vi "fpga_LP2ControlUnit (M Class_60Hz).vi"(0 "#Ch":fxp<+,5,5>=16.0, 1 "reset":bool, 2 "input valid":bool) -> (5 "ready for input":bool, 7 "output valid":bool, 8 "opState":T1, 9 "coefRDAddr":fxp<+,11,11>)   [LabVIEW 2013, in "NI_EP_PMU_FPGA.lvlib"]
uses:
  <vilib>/addons/Electrical Power/PMU/NI_EP_PMU_FPGA.lvlib
  <vilib>/rvi/FXPMathLib/basic elements/FxpAddSub/XNode/nifxpmath_AddSub.xnode
  <vilib>/rvi/FXPMathLib/sim/FxpSim.dll
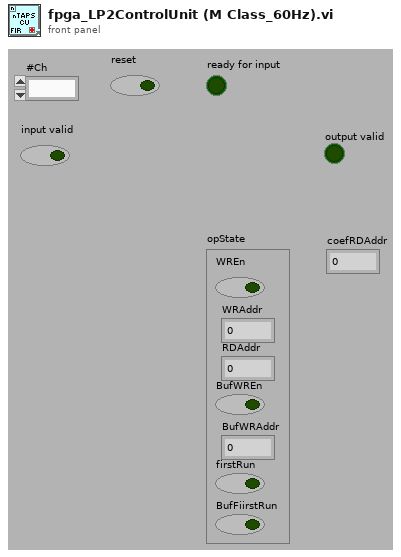
[diagram p1: front panel]
types:
  T1 = cluster{"WREn":bool, "WRAddr":fxp<+,15,15>, "RDAddr":fxp<+,15,15>, "BufWREn":bool, "BufWRAddr":fxp<+,15,15>, "firstRun":bool, "BufFiirstRun":bool}
  T2 = cluster{"idle":bool, "ready for input":bool, "macWrap":bool, "inputBufWRAddr":fxp<+,15,15>, "coefRDAddr":fxp<+,11,11>, "stateMemRDAddr":fxp<+,15,15>, "stateMemPageRDAddr":fxp<+,15,15>, "chCnt":fxp<+,5,5>, "first run?":bool, "firstRunCnt":fxp<+,15,15>, "buf first run?":bool, "bufFirstRunCnt":fxp<+,15,15>}
  T3 = cluster{"inputBufWRAddr":fxp<+,15,15>, "coefRDAddr":fxp<+,11,11>, "stateMemPageRDAddr":fxp<+,15,15>, "#Ch*(#TPPM-1)-1":fxp<+,15,15>, "#Ch*(#TPPM-2)-1":fxp<+,15,15>, "#Ch*#BufSize":fxp<+,15,15>, "2*#Ch-1":fxp<+,5,5>, "-#Ch":fxp<+,15,15>}
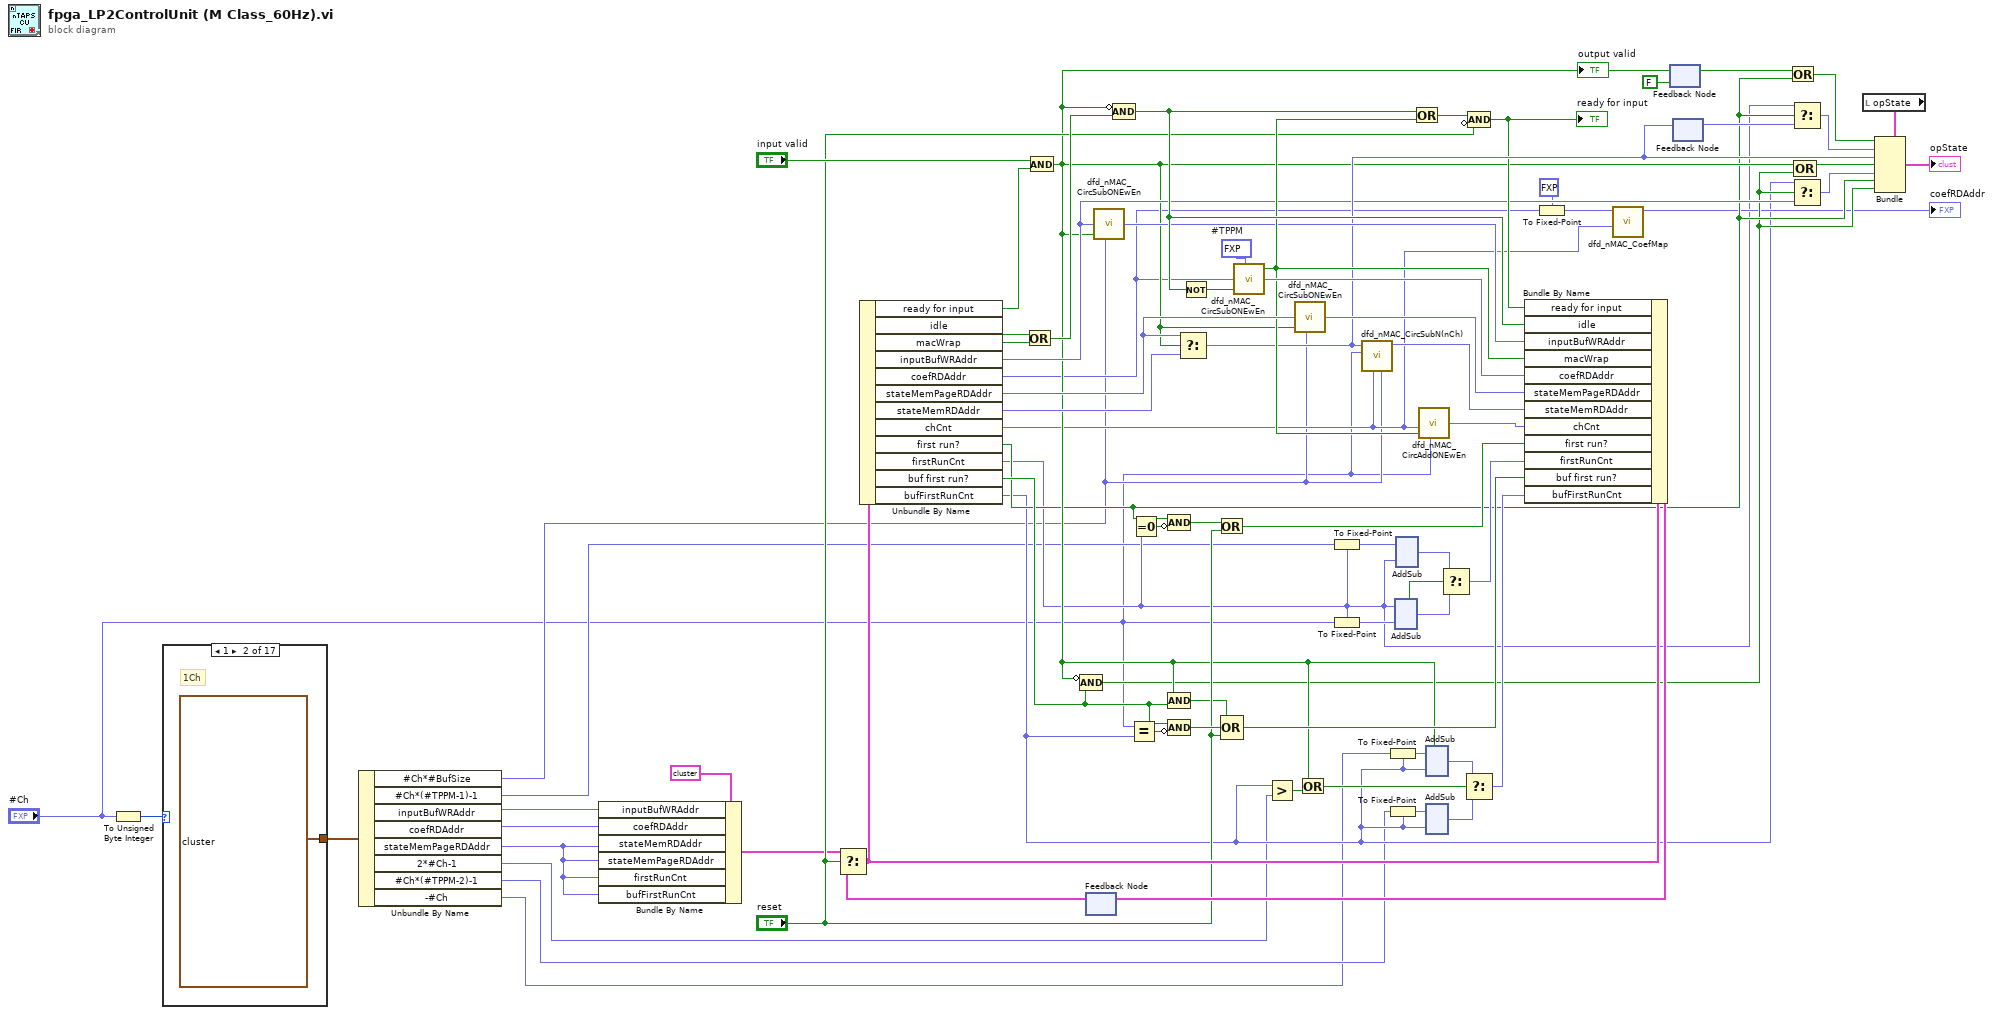
[diagram p0: block diagram]
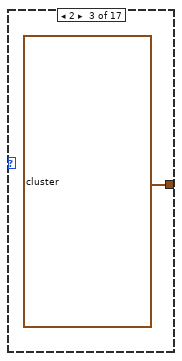
[diagram p3: hidden frame]
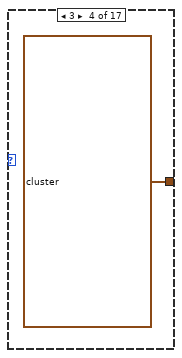
[diagram p4: hidden frame]
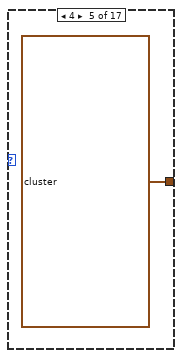
[diagram p5: hidden frame]
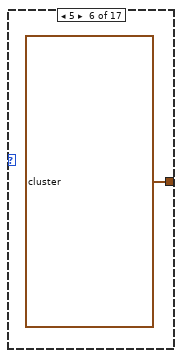
[diagram p6: hidden frame]
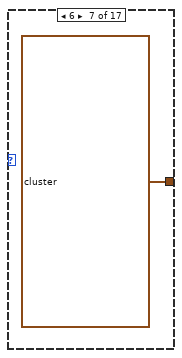
[diagram p7: hidden frame]
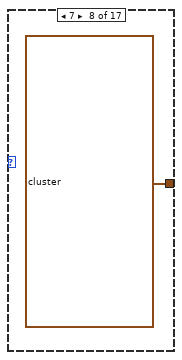
[diagram p8: hidden frame]
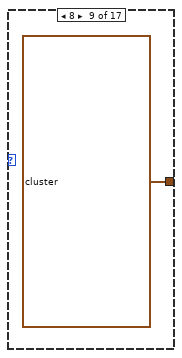
[diagram p9: hidden frame]
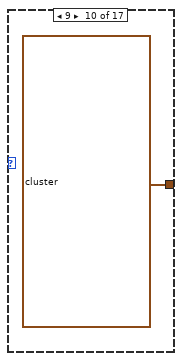
[diagram p10: hidden frame]
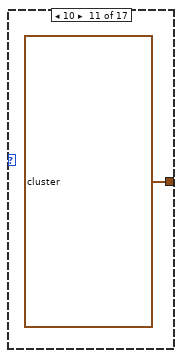
[diagram p11: hidden frame]
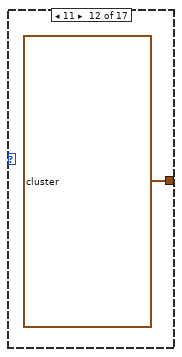
[diagram p12: hidden frame]
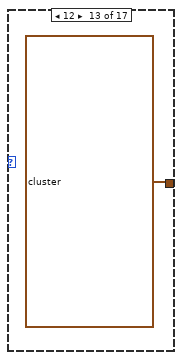
[diagram p13: hidden frame]
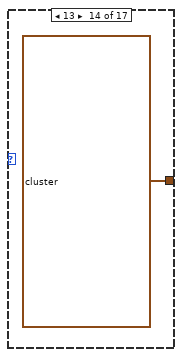
[diagram p14: hidden frame]
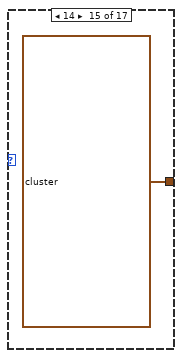
[diagram p15: hidden frame]
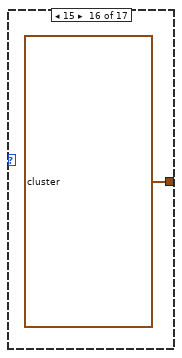
[diagram p16: hidden frame]
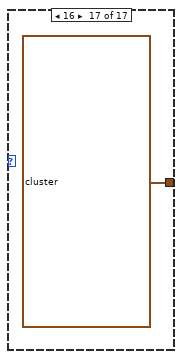
[diagram p17: hidden frame]
diagram:
  w68 = fxp<+,11,11> 1188.0  # #TPPM
  n1 = To Unsigned Byte Integer(number="#Ch") -> (unsigned 8bit integer=w13:u8)
  n2 = case shown="1" w13 {
    tunnel: [_ T3 {"inputBufWRAddr"=0.0, "coefRDAddr"=1187.0, "stateMemPageRDAddr"=1187.0, "#Ch*(#TPPM-1)-1"=1186.0, "#Ch*(#TPPM-2)-1"=1185.0, "#Ch*#BufSize"=1188.0, "2*#Ch-1"=1.0, "-#Ch"=32767.0} ("Cluster") T3 {"inputBufWRAddr"=1.0, "coefRDAddr"=1187.0, "stateMemPageRDAddr"=2375.0, "#Ch*(#TPPM-1)-1"=2373.0, "#Ch*(#TPPM-2)-1"=2371.0, "#Ch*#BufSize"=2376.0, "2*#Ch-1"=3.0, "-#Ch"=32766.0} ("Cluster") T3 {"inputBufWRAddr"=2.0, "coefRDAddr"=1187.0, "stateMemPageRDAddr"=3563.0, "#Ch*(#TPPM-1)-1"=3560.0, "#Ch*(#TPPM-2)-1"=3557.0, "#Ch*#BufSize"=3564.0, "2*#Ch-1"=5.0, "-#Ch"=32765.0} ("Cluster") T3 {"inputBufWRAddr"=3.0, "coefRDAddr"=1187.0, "stateMemPageRDAddr"=4751.0, "#Ch*(#TPPM-1)-1"=4747.0, "#Ch*(#TPPM-2)-1"=4743.0, "#Ch*#BufSize"=4752.0, "2*#Ch-1"=7.0, "-#Ch"=32764.0} ("Cluster") T3 {"inputBufWRAddr"=4.0, "coefRDAddr"=1187.0, "stateMemPageRDAddr"=5939.0, "#Ch*(#TPPM-1)-1"=5934.0, "#Ch*(#TPPM-2)-1"=5929.0, "#Ch*#BufSize"=5940.0, "2*#Ch-1"=9.0, "-#Ch"=32763.0} ("Cluster") T3 {"inputBufWRAddr"=5.0, "coefRDAddr"=1187.0, "stateMemPageRDAddr"=7127.0, "#Ch*(#TPPM-1)-1"=7121.0, "#Ch*(#TPPM-2)-1"=7115.0, "#Ch*#BufSize"=7128.0, "2*#Ch-1"=11.0, "-#Ch"=32762.0} ("Cluster") T3 {"inputBufWRAddr"=6.0, "coefRDAddr"=1187.0, "stateMemPageRDAddr"=8315.0, "#Ch*(#TPPM-1)-1"=8308.0, "#Ch*(#TPPM-2)-1"=8301.0, "#Ch*#BufSize"=8316.0, "2*#Ch-1"=13.0, "-#Ch"=32761.0} ("Cluster") T3 {"inputBufWRAddr"=7.0, "coefRDAddr"=1187.0, "stateMemPageRDAddr"=9503.0, "#Ch*(#TPPM-1)-1"=9495.0, "#Ch*(#TPPM-2)-1"=9487.0, "#Ch*#BufSize"=9504.0, "2*#Ch-1"=15.0, "-#Ch"=32760.0} ("Cluster") T3 {"inputBufWRAddr"=8.0, "coefRDAddr"=1187.0, "stateMemPageRDAddr"=10691.0, "#Ch*(#TPPM-1)-1"=10682.0, "#Ch*(#TPPM-2)-1"=10673.0, "#Ch*#BufSize"=10692.0, "2*#Ch-1"=17.0, "-#Ch"=32759.0} ("Cluster") T3 {"inputBufWRAddr"=9.0, "coefRDAddr"=1187.0, "stateMemPageRDAddr"=11879.0, "#Ch*(#TPPM-1)-1"=11869.0, "#Ch*(#TPPM-2)-1"=11859.0, "#Ch*#BufSize"=11880.0, "2*#Ch-1"=19.0, "-#Ch"=32758.0} ("Cluster") T3 {"inputBufWRAddr"=10.0, "coefRDAddr"=1187.0, "stateMemPageRDAddr"=13067.0, "#Ch*(#TPPM-1)-1"=13056.0, "#Ch*(#TPPM-2)-1"=13045.0, "#Ch*#BufSize"=13068.0, "2*#Ch-1"=21.0, "-#Ch"=32757.0} ("Cluster") T3 {"inputBufWRAddr"=11.0, "coefRDAddr"=1187.0, "stateMemPageRDAddr"=14255.0, "#Ch*(#TPPM-1)-1"=14243.0, "#Ch*(#TPPM-2)-1"=14231.0, "#Ch*#BufSize"=14256.0, "2*#Ch-1"=23.0, "-#Ch"=32756.0} ("Cluster") T3 {"inputBufWRAddr"=12.0, "coefRDAddr"=1187.0, "stateMemPageRDAddr"=15443.0, "#Ch*(#TPPM-1)-1"=15430.0, "#Ch*(#TPPM-2)-1"=15417.0, "#Ch*#BufSize"=15444.0, "2*#Ch-1"=25.0, "-#Ch"=32755.0} ("Cluster") T3 {"inputBufWRAddr"=13.0, "coefRDAddr"=1187.0, "stateMemPageRDAddr"=16631.0, "#Ch*(#TPPM-1)-1"=16617.0, "#Ch*(#TPPM-2)-1"=16603.0, "#Ch*#BufSize"=16632.0, "2*#Ch-1"=27.0, "-#Ch"=32754.0} ("Cluster") T3 {"inputBufWRAddr"=14.0, "coefRDAddr"=1187.0, "stateMemPageRDAddr"=17819.0, "#Ch*(#TPPM-1)-1"=17804.0, "#Ch*(#TPPM-2)-1"=17789.0, "#Ch*#BufSize"=17820.0, "2*#Ch-1"=29.0, "-#Ch"=32753.0} ("Cluster") T3 {"inputBufWRAddr"=15.0, "coefRDAddr"=1187.0, "stateMemPageRDAddr"=19007.0, "#Ch*(#TPPM-1)-1"=18991.0, "#Ch*(#TPPM-2)-1"=18975.0, "#Ch*#BufSize"=19008.0, "2*#Ch-1"=31.0, "-#Ch"=32752.0} ("Cluster")] -> w12
    frame 0, Default {
    }
    frame 1 {
      # "1Ch"
    }
    frame 2 {
    }
    frame 3 {
    }
    frame 4 {
    }
    frame 5 {
    }
    frame 6 {
    }
    frame 7 {
    }
    frame 8 {
    }
    frame 9 {
    }
    frame 10 {
    }
    frame 11 {
    }
    frame 12 {
    }
    frame 13 {
    }
    frame 14 {
    }
    frame 15 {
    }
    frame 16 {
    }
  }
  n3 = Unbundle By Name(w12) -> ("#Ch*#BufSize"=w6:fxp<+,15,15>, "#Ch*(#TPPM-1)-1"=w5:fxp<+,15,15>, "inputBufWRAddr"=w11:fxp<+,15,15>, "coefRDAddr"=w10:fxp<+,11,11>, "stateMemPageRDAddr"=w9:fxp<+,15,15>, "2*#Ch-1"=w4:fxp<+,5,5>, "#Ch*(#TPPM-2)-1"=w3:fxp<+,15,15>, "-#Ch"=w2:fxp<+,15,15>)
  n4 = Bundle By Name(cluster=T2 {"idle"=TRUE, "ready for input"=FALSE, "macWrap"=FALSE, "inputBufWRAddr"=15.0, "coefRDAddr"=1187.0, "stateMemRDAddr"=19007.0, "stateMemPageRDAddr"=19007.0, "chCnt"=0.0, "first run?"=TRUE, "firstRunCnt"=19007.0, "buf first run?"=TRUE, "bufFirstRunCnt"=19007.0} ("CUInitialState"), "inputBufWRAddr"=w11, "coefRDAddr"=w10, "stateMemRDAddr"=w9, "stateMemPageRDAddr"=w9, "firstRunCnt"=w9, "bufFirstRunCnt"=w9) -> (w7:T2)
  n5 = feedback #1() -> (w69:T2)  [unwired: 1 out]
  n6 = Select(t=w7, s="reset", f=w69) -> (s? t:f=w66:T2)
  n7 = Unbundle By Name(w66) -> ("ready for input"=w64:bool, "idle"=w56:bool, "macWrap"=w57:bool, "inputBufWRAddr"=w43:fxp<+,15,15>, "coefRDAddr"=w21:fxp<+,11,11>, "stateMemPageRDAddr"=w72:fxp<+,15,15>, "stateMemRDAddr"=w73:fxp<+,15,15>, "chCnt"=w23:fxp<+,5,5>, "first run?"=w26:bool, "firstRunCnt"=w17:fxp<+,15,15>, "buf first run?"=w29:bool, "bufFirstRunCnt"=w14:fxp<+,15,15>)
  n8 = Or(x=w56, y=w57) -> (x .or. y?=w63:bool)
  n9 = And(x="input valid", y=w64) -> (x .and. y?=w28:bool)
  "output valid" <- w28
  n10 = Compound Arithmetic op=AND(invert w28, w29) -> (w25:bool)
  n11 = call "dfd_nMAC_CircSubONEwEn.vi"("len"=w6, "idxIn"=w43, "Enable"=w28) -> ("idxOut"=w59:fxp<+,15,15>)  [unwired: 5 in, 1 out]
  n12 = Compound Arithmetic op=AND(invert w28, w63) -> (w62:bool)
  n13 = Equal?(x="#Ch", y=w14) -> (x = y?=w54:bool)
  n14 = Equal To 0?(x=w17) -> (x = 0?=w38:bool)
  n15 = Compound Arithmetic op=AND(w26, invert w38) -> (w39:bool)
  n16 = Compound Arithmetic op=AND(w28, w29) -> (w27:bool)
  n17 = Compound Arithmetic op=AND(w29, invert w54) -> (w53:bool)
  n18 = Select(t=w72, s=w28, f=w73) -> (s? t:f=w58:fxp<+,15,15>)
  n19 = Not(x=w62) -> (.not. x?=w70:bool)
  n20 = Or(x=w39, y="reset") -> (x .or. y?=w35:bool)
  n21 = Compound Arithmetic op=OR(w27, w53, "reset") -> (w33:bool)
  n22 = call "dfd_nMAC_CircSubONEwEn.vi"("len"=w68, "idxIn"=w21, "Enable"=w70) -> ("wrap?"=w60:bool, "idxOut"=w75:fxp<+,11,11>)  [unwired: 5 in]
  n23 = Greater?(x=w14, y=w4) -> (0:w37:bool)
  n24 = call "dfd_nMAC_CircSubONEwEn.vi"("len"=w6, "idxIn"=w72, "Enable"=w28) -> ("idxOut"=w74:fxp<+,15,15>)  [unwired: 5 in, 1 out]
  n25 = Or(x=w28, y=w37) -> (x .or. y?=w36:bool)
  n26 = To Fixed-Point(fixed-point type=w17, number=w5) -> (fixed-point=w19:fxp<+,15,15>)
  n27 = To Fixed-Point(fixed-point type=w17, number="#Ch") -> (fixed-point=w18:fxp<+,15,15>)
  n28 = call "dfd_nMAC_CircSubN(nCh).vi"("bufSize*#ch"=w6, "curChIdx"=w23, "#ch"="#Ch", "idxIn"=w58) -> ("idxOut"=w77:fxp<+,15,15>)  [unwired: 7 in]
  n29 = To Fixed-Point(fixed-point type=w14, number=w2) -> (fixed-point=w16:fxp<+,15,15>)
  n30 = To Fixed-Point(fixed-point type=w14, number=w3) -> (fixed-point=w15:fxp<+,15,15>)
  n31 = xnode ("AddSub")("x"=w17, "y"=w18) -> ("s"=w42:fxp<+,15,15>, "borrow-out"=w41:bool)
  n32 = xnode ("AddSub")("x"=w19, "y"=w17) -> ("s"=w40:fxp<+,15,15>)  [unwired: 1 out]
  n33 = Or(x=w62, y=w60) -> (x .or. y?=w61:bool)
  n34 = call "dfd_nMAC_CircAddONEwEn.vi"("len"="#Ch", "idxIn"=w23, "Enable"=w60) -> ("idxOut"=w76:fxp<+,5,5>)  [unwired: 5 in, 1 out]
  n35 = xnode ("AddSub")("x"=w16, "y"=w14, "use zero instead of x"=w28) -> ("s"=w50:fxp<+,15,15>)  [unwired: 1 out]
  n36 = xnode ("AddSub")("x"=w15, "y"=w14) -> ("s"=w51:fxp<+,15,15>)  [unwired: 1 out]
  n37 = Select(t=w40, s=w41, f=w42) -> (s? t:f=w34:fxp<+,15,15>)
  n38 = Select(t=w50, s=w36, f=w51) -> (s? t:f=w32:fxp<+,15,15>)
  n39 = Compound Arithmetic op=AND(w61, invert "reset") -> (w55:bool)
  "ready for input" <- w55
  n40 = Bundle By Name(cluster=w66, "ready for input"=w55, "idle"=w62, "inputBufWRAddr"=w59, "macWrap"=w60, "coefRDAddr"=w75, "stateMemPageRDAddr"=w74, "stateMemRDAddr"=w77, "chCnt"=w76, "first run?"=w35, "firstRunCnt"=w34, "buf first run?"=w33, "bufFirstRunCnt"=w32) -> (w67:T2)
  n41 = feedback-in #1(w67) -> ()
  n42 = To Fixed-Point(fixed-point type=fxp<+,11,11> 0.0 ("CoefAddr"), number=w21) -> (fixed-point=w22:fxp<+,11,11>)
  n43 = call "dfd_nMAC_CoefMap.vi"("chCnt"=w23, "coefOffsetAddr"=w22) -> ("coefRDAddr"=→"coefRDAddr":fxp<+,11,11>)  [unwired: 9 in]
  n44 = feedback-in #2(w28) -> ()
  n45 = feedback #2(FALSE) -> (w49:bool)
  n46 = feedback-in #3(w58) -> ()
  n47 = feedback #3() -> (w47:fxp<+,15,15>)  [unwired: 1 out]
  n48 = Or(x=w49, y=w26) -> (x .or. y?=w48:bool)
  n49 = Select(t=w17, s=w26, f=w47) -> (s? t:f=w46:fxp<+,15,15>)
  n50 = Select(t=w14, s=w25, f=w43) -> (s? t:f=w45:fxp<+,15,15>)
  n51 = Compound Arithmetic op=OR(w28, w25) -> (w44:bool)
  n52 = local read "opState"() -> (w30:T1)
  n53 = Bundle(cluster=w30, "WREn"=w48, "WRAddr"=w46, "RDAddr"=w58, "BufWREn"=w44, "BufWRAddr"=w45, "firstRun"=w26, "BufFiirstRun"=w25) -> (→"opState":T1)
